vi "Set and Get with MathCAD.vi"() -> ()   [LabVIEW 2015, in "AguaClara Library.lvlib"]
doc: "This VI uses native LabVIEW and Mathcad functions to write to and read from files containing large blocks of data. For large datasets, typically this is a much faster approach to send data between LabVIEW and Mathcad. However, native functions used in the example could be used in conjunction with the other VIs contained in the Mathcad Connectivity Toolkit to send via ActiveX other variables such as filename or location of file."
uses:
  AguaClara Library.lvlib
  mathcad/Easy/MathCad_Easy_String_Set_Var.vi
  mathcad/Easy/MathCad_Easy_Numeric_Get_Var.vi
  mathcad/Easy/MathCad_Easy_Matrix_Get_2D.vi
  mathcad/Easy/MathCad_Easy_Numeric_Set_Var.vi
panel:
  out "Array":dbl[][](array[numeric]) format="%.2f"
  out "value":dbl format="%.2f"
  in  "MathCAD file path":path=path "C:/Documents and Settings/All Users/Documents/AguaClara LabVIEW/mathcad/File IO with LabVIEW.xmcd"
  in  "stop":bool
  in  "Recieve":bool
  in  "Send":bool
  in  "Data Path (Send to Mathcad)":path=path "C:/Documents and Settings/All Users/Documents/AguaClara LabVIEW/Data File.PRN"
  in  "Send 2D array  to Mathcad":sgl[][](array[numeric])=[[1.0, 2.0, 2.0, 475.85], [5.6, 6.0, 5.5, 589.0], [5.563, 5.56, 2.0, 53.65], [9.58, 53.5, 0.0, 53.5]] format="%.3f"
  # "This VI sends an array to a File that Mathcad's READPRN() function can read. The Mathcad worksheet that is called send the data to another file via the WRITEPRN() function. LabVIEW reads the path information from Mathcad and retrieves the data."
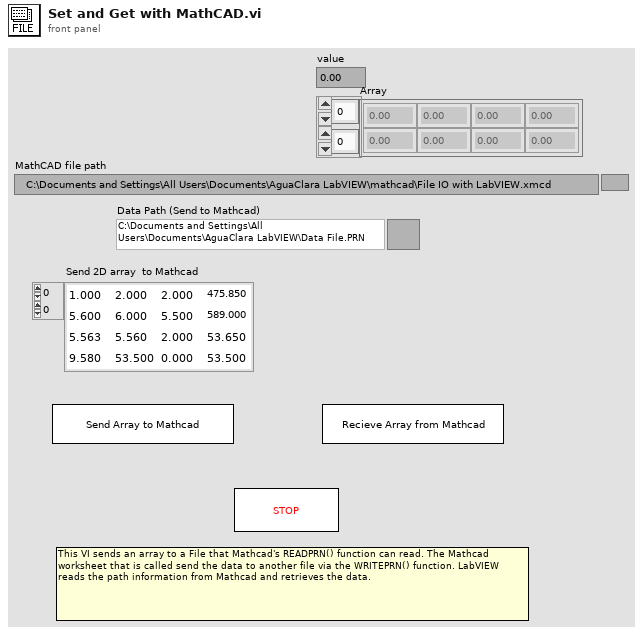
[diagram p1: front panel]
types:
  T1 = typedef "Mathcad Reference.ctl" = cluster{"Application Reference":refnum<k7>, "Worksheets Reference":refnum<k7>, " Worksheet Reference":refnum<k7>}
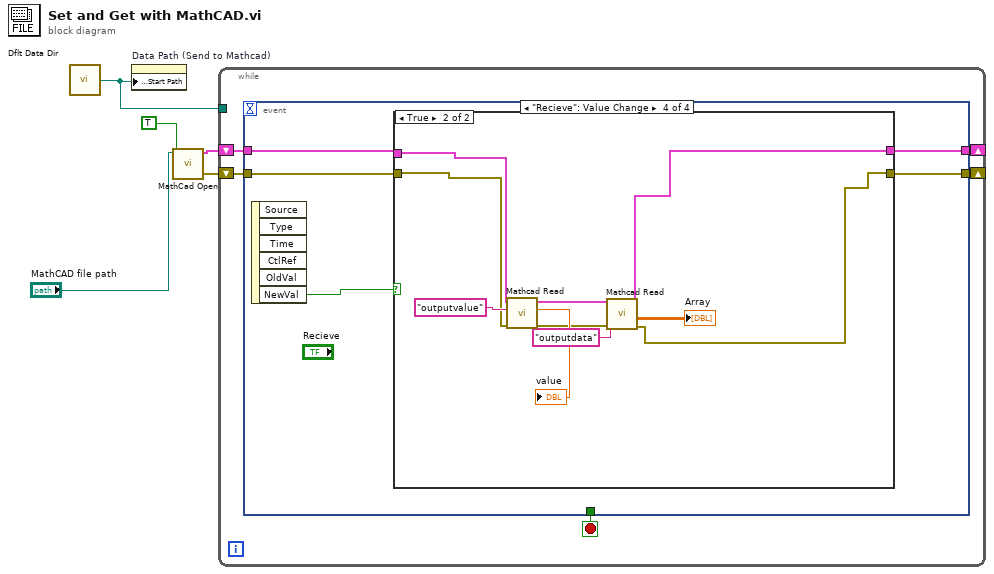
[diagram p0: block diagram]
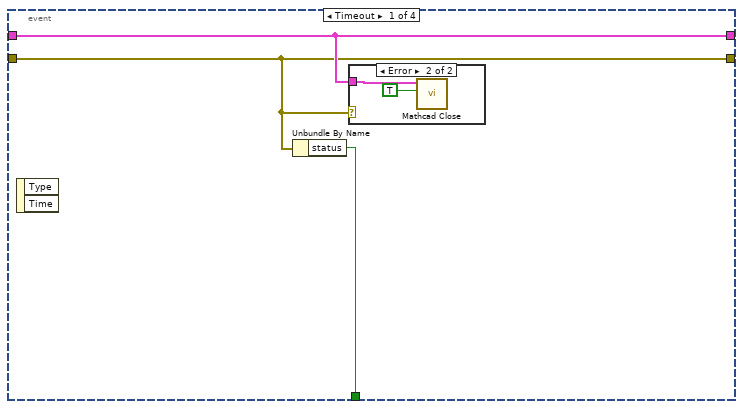
[diagram p2: hidden frame]
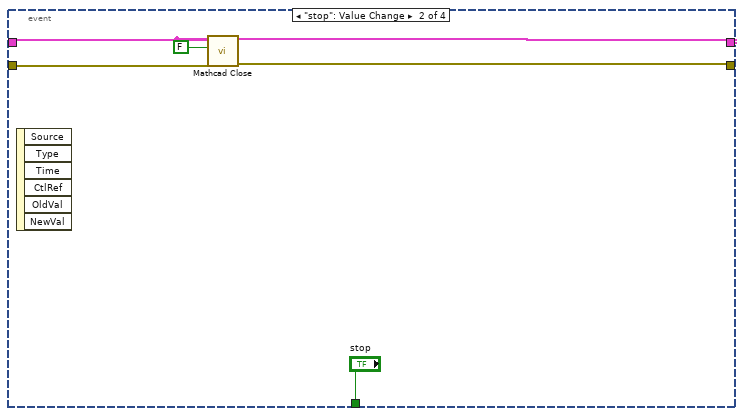
[diagram p4: hidden frame]
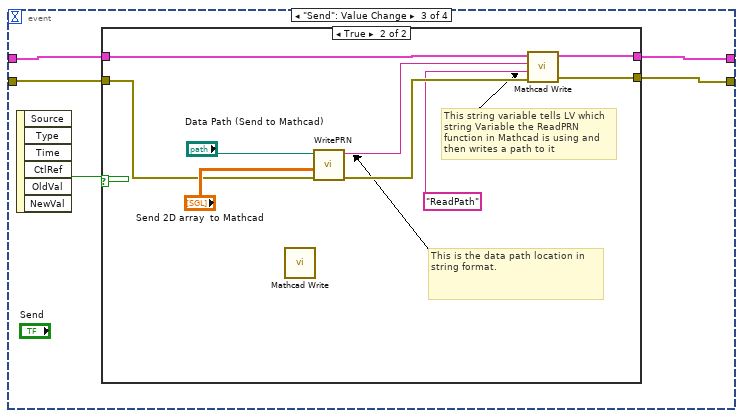
[diagram p5: hidden frame]
diagram:
  n1 = call <vilib>:"Dflt Data Dir.vi"() -> ("App:Default Data Directory"=w2:path)
  n2 = property on="Data Path (Send to Mathcad)" class="Path"("Browse Options:Start Path"=w2) -> ()  [unwired: 2 in, 2 out]
  n3 = call "MathCad Open.vi"("Visible"=TRUE, "File Path"="MathCAD file path") -> ("error out (no error)"=w4:errorcluster, "Mathcad Reference"=w3:T1)  [unwired: 8 in]
  n4 = while {
    shift-right: [w8] -> _
    shift-left: w4 -> [w9]
    shift-right: [w7] -> _
    shift-left: w3 -> [w6]
    tunnel: w2 -> [_]
    stop <- w10 stop-if-true
    n5 = event shown="[3] \"Recieve\": Value Change" {
      selector: _ -> [_ _ _ _]
      dyn-events: _ -> [_ _ _ _]
      timeout: _ -> [_ _ _ _]
      tunnel: [w11 "stop" _ _] -> w10
      tunnel: w9 -> [w12 w19 w24 w37]
      tunnel: [w12 w17 w21 w38] -> w8
      tunnel: [w13 w16 w22 w39] -> w7
      tunnel: w6 -> [w13 w16 w23 w40]
      event Timeout {
        n6 = event-data() -> ()  [unwired: 1 in, 2 out]
        n7 = Unbundle By Name(w12) -> ("status"=w11:bool)
        n8 = case shown="Error" w12 {
          tunnel: w13 -> [_ w15]
          frame No Error {
          }
          frame Error {
            n9 = call "Mathcad Close.vi"("Exit Mathcad?"=TRUE, "Mathcad Reference"=w15) -> ()  [unwired: 9 in, 1 out]
          }
        }
      }
      event "stop": Value Change {
        n10 = event-data() -> ()  [unwired: 1 in, 6 out]
        n11 = call "Mathcad Close.vi"("Error In"=w19, "Exit Mathcad?"=FALSE, "Mathcad Reference"=w16) -> ("Error Out"=w17:errorcluster)  [unwired: 8 in]
      }
      event "Send": Value Change {
        n12 = event-data() -> ("NewVal"=w25:bool)  [unwired: 1 in, 5 out]
        n13 = case shown="True" w25 {
          tunnel: w24 -> [w26 w30]
          tunnel: w23 -> [w27 w35]
          tunnel: [w27 w34] -> w22
          tunnel: [w26 w33] -> w21
          frame False {
          }
          frame True {
            # "This is the data path location in string format."
            # "This string variable tells LV which string Variable the ReadPRN function in Mathcad is using and then writes a path to it"
            n14 = call-poly "Mathcad Write.vi"() -> ()  [unwired: 10 in, 2 out]
            n15 = call "WritePRN.vi"("error in (no error)"=w30, "2D Data"="Send 2D array  to Mathcad", "Data Path (Send to Mathcad)"="Data Path (Send to Mathcad)") -> ("error out"=w29:errorcluster, "Data Path(String)"=w31:string)  [unwired: 7 in]
            n16 = call-poly "Mathcad Write.vi"("error in (no error)"=w29, "Variable Name"="ReadPath" ("New Variable Name"), "String Value"=w31, "Mathcad Reference"=w35) -> ("error out"=w33:errorcluster, "Mathcad Reference"=w34:T1)  [unwired: 6 in]
          }
        }
      }
      event "Recieve": Value Change {
        n17 = event-data() -> ("NewVal"=w41:bool)  [unwired: 1 in, 5 out]
        n18 = case shown="True" w41 {
          tunnel: [w42 w44] -> w39
          tunnel: w40 -> [w42 w51]
          tunnel: w37 -> [w43 w50]
          tunnel: [w43 w45] -> w38
          frame False {
          }
          frame True {
            n19 = call-poly "Mathcad Read.vi"("error in (no error)"=w50, "Variable  Name"="outputvalue", "Mathcad Reference"=w51) -> ("error out"=w48:errorcluster, "value"=→"value":dbl, "Mathcad Reference"=w49:T1)  [unwired: 6 in]
            n20 = call-poly "Mathcad Read.vi"("error in (no error)"=w48, "Variable  Name"="outputdata", "Mathcad Reference"=w49) -> ("error out"=w45:errorcluster, "Array"=→"Array":dbl[][], "Mathcad Reference"=w44:T1)  [unwired: 6 in]
          }
        }
      }
    }
  }
